vi "The_Regulators.vi"() -> (0 "Error Out":errorcluster, 3 "DAQmx Task Name":refnum<k21>)   [LabVIEW 2014]
uses:
  <vilib>/DAQmx/create/channels.llb/DAQmx Create Channel (AI-Voltage-Basic).vi
panel:
  in  "Channel":tag
  in  "Min V":dbl=-5.0 format="%0.2f"
  in  "Max V":dbl=5.0 format="%0.2f"
  in  "Channel":tag
  in  "Max V":dbl=5.0 format="%0.2f"
  in  "Min V":dbl=-5.0 format="%0.2f"
  in  "Error In":errorcluster
  # "The Regulators\n\nConsists of 2 Inputs\n\n( The Bottom, and the Top Regulator )"
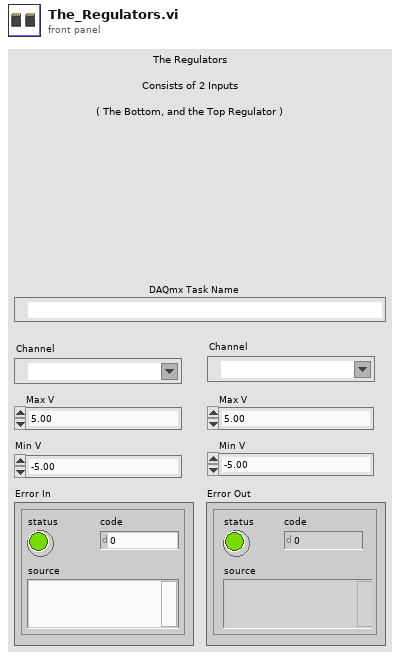
[diagram p1: front panel]
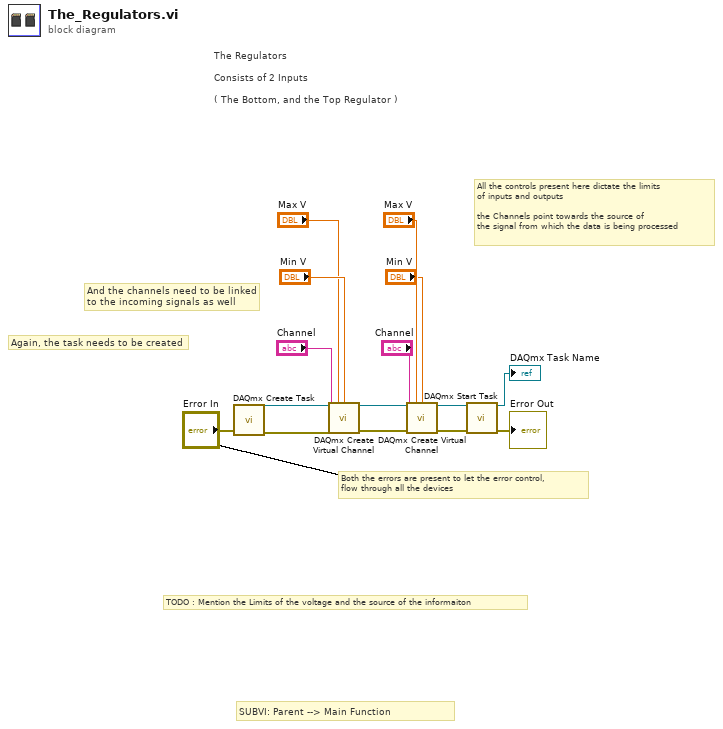
[diagram p0: block diagram]
diagram:
  # "SUBVI: Parent --> Main Function"
  # "TODO : Mention the Limits of the voltage and the source of the informaiton"
  # "All the controls present here dictate the limits \nof inputs and outputs \n\nthe Channels point towards the source of \nthe signal from which the data is being processed"
  # "Both the errors are present to let the error control,\nflow through all the devices"
  # "And the channels need to be linked \nto the incoming signals as well"
  # "Again, the task needs to be created"
  # "The Regulators\n\nConsists of 2 Inputs\n\n( The Bottom, and the Top Regulator )"
  n1 = call <vilib>:"DAQmx Create Task.vi"("error in"="Error In") -> ("task out"=w3:refnum<k21>, "error out"=w2:errorcluster)  [unwired: 13 in]
  n2 = call-poly <vilib>:"DAQmx Create Virtual Channel.vi"("task in"=w3, "maximum value"="Max V", "minimum value"="Min V", "physical channels"="Channel", "error in"=w2) -> ("task out"=w15:refnum<k21>, "error out"=w14:errorcluster)  [unwired: 9 in]
  n3 = call-poly <vilib>:"DAQmx Create Virtual Channel.vi"("task in"=w15, "maximum value"="Max V", "minimum value"="Min V", "physical channels"="Channel", "error in"=w14) -> ("task out"=w13:refnum<k21>, "error out"=w12:errorcluster)  [unwired: 9 in]
  n4 = call <vilib>:"DAQmx Start Task.vi"("task/channels in"=w13, "error in"=w12) -> ("task out"=→"DAQmx Task Name":refnum<k21>, "error out"=→"Error Out":errorcluster)  [unwired: 12 in]
